vi "chaosui-default-decode.vi"(8 "JSON string":string) -> (0 "parse_error":i32, 1 "dev_error":bool, 2 "dev_state":T1, 3 "timestamp":u64, 4 "dev_error_status":string)   [LabVIEW 2014]
uses:
  ChaosDevState.ctl
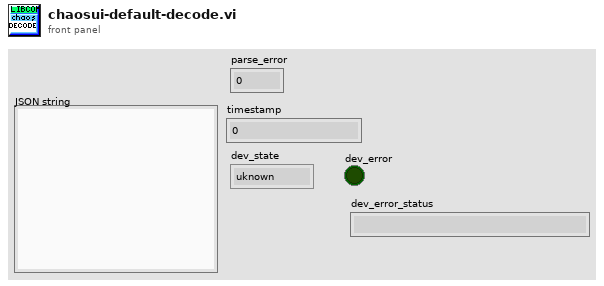
[diagram p1: front panel]
types:
  T1 = typedef "ChaosDevState.ctl" = enum16{"uknown", "stop", "init", "deinit", "start"}
  T2 = cluster{"error_status":string, "log_status":string, "dev_status":string}
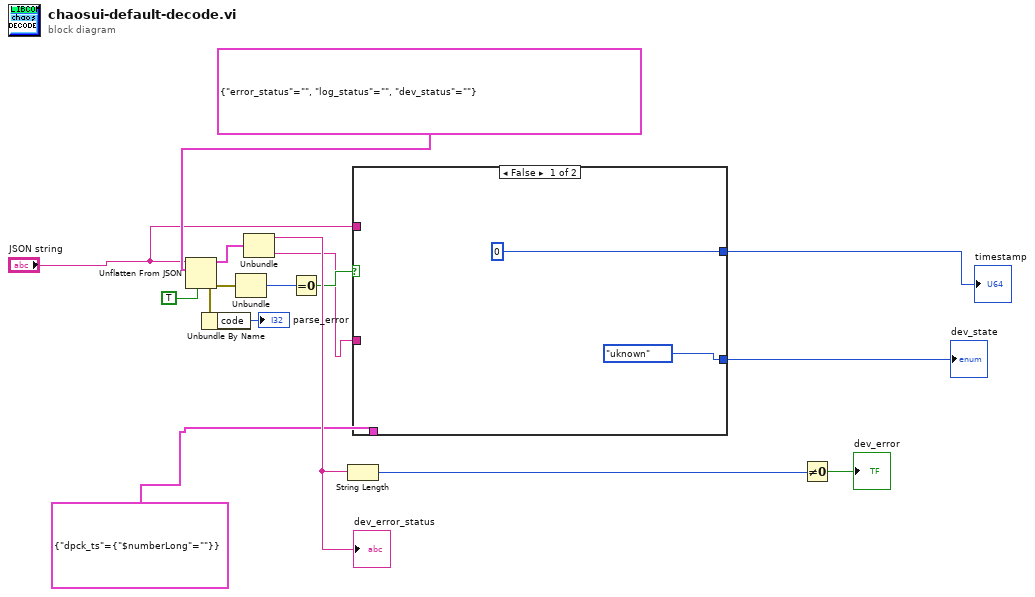
[diagram p0: block diagram]
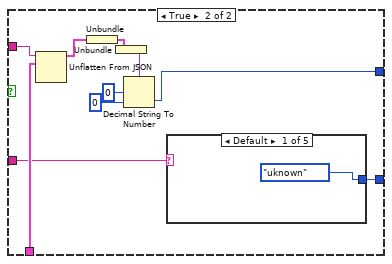
[diagram p2: hidden frame]
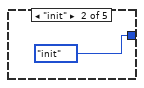
[diagram p3: hidden frame]
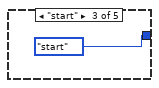
[diagram p4: hidden frame]
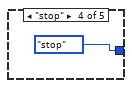
[diagram p5: hidden frame]
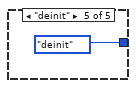
[diagram p6: hidden frame]
diagram:
  n1 = Unflatten From JSON(JSON string="JSON string", type and defaults=T2 {"error_status"="", "log_status"="", "dev_status"=""}, default null elements? (F)=TRUE) -> (value=w14:T2, error out=w13:errorcluster)  [unwired: 4 in]
  n2 = Unbundle By Name(w13) -> ("code"=→"parse_error":i32)
  n3 = Unbundle(w13) -> ("code"=w15:i32)  [unwired: 2 out]
  n4 = Unbundle(w14) -> ("error_status"=w7:string, "dev_status"=w2:string)  [unwired: 1 out]
  "dev_error_status" <- w7
  n5 = Equal To 0?(x=w15) -> (x = 0?=w6:bool)
  n6 = String Length(string=w7) -> (length=w12:i32)
  n7 = case shown="False" w6 {
    tunnel: "JSON string" -> [_ w27]
    tunnel: cluster{"dpck_ts":cluster{"$numberLong":string}} {"dpck_ts"={"$numberLong"=""}} -> [_ w26]
    tunnel: [u64 0 w21] -> w3
    tunnel: w2 -> [_ w19]
    tunnel: [ChaosDevState."uknown" ("dev_state") w18] -> w1
    frame False {
    }
    frame True {
      n8 = Unflatten From JSON(JSON string=w27, type and defaults=w26) -> (value=w25:cluster{"dpck_ts":cluster{"$numberLong":string}})  [unwired: 5 in, 1 out]
      n9 = Unbundle(w25) -> ("dpck_ts"=w24:cluster{"$numberLong":string})
      n10 = Unbundle(w24) -> ("$numberLong"=w20:string)
      n11 = Decimal String To Number(string=w20, offset=0, default (0L)=u64 0 ("default (0 I32)")) -> (number=w21:u64)  [unwired: 1 out]
      n12 = case shown="Default" w19 {
        tunnel: [ChaosDevState."uknown" ("dev_state") ChaosDevState."init" ("dev_state") ChaosDevState."start" ("dev_state") ChaosDevState."stop" ("dev_state") ChaosDevState."deinit" ("dev_state")] -> w18
        frame Default {
        }
        frame "init" {
        }
        frame "start" {
        }
        frame "stop" {
        }
        frame "deinit" {
        }
      }
    }
  }
  "timestamp" <- w3
  "dev_state" <- w1
  n13 = Not Equal To 0?(x=w12) -> (x != 0?=→"dev_error":bool)
